vi "Unflatten Value.vi"(0 "String In":refnum<class "String.lvclass">, 7 "Value":string, 11 "Error In":errorcluster) -> (4 "String Out":refnum<class "String.lvclass">, 15 "Error Out":errorcluster)   [LabVIEW 2016, in "String.lvclass"]
uses:
  String.lvclass
  String.lvclass/String.ctl
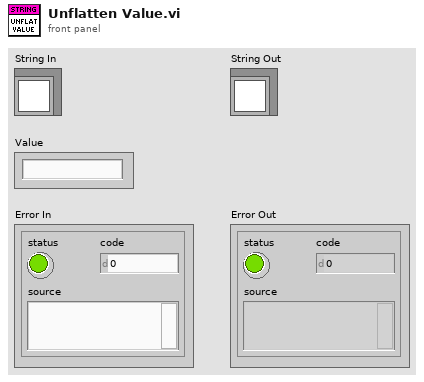
[diagram p1: front panel]
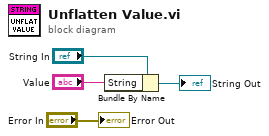
[diagram p0: block diagram]
diagram:
  n1 = Bundle By Name(cluster="String In", "String"="Value") -> (→"String Out":refnum<class "String.lvclass">)
  "Error Out" <- "Error In"
